vi "Strip prefix.vi"(10 "prefix":i32, 11 "address":refnum<class "IPv4 Network Address.lvclass">) -> (2 "subnet address":refnum<class "IPv4 Network Address.lvclass">)   [LabVIEW 2020, in "NI_WFCN.lvlib" / "IPv4 Network Address.lvclass"]
doc: "Masks the prefix off of this address, producing the subnet address. For instance, given address 192.168.1.2 and prefix 16, return 192.168.0.0."
uses:
  <vilib>/net/WFCN/Addressing/IPv4 Network Address/IPv4 Network Address.lvclass
  <vilib>/net/WFCN/Addressing/IPv4 Network Address/IPv4 Network Address.lvclass/IPv4 Network Address.ctl
  <vilib>/net/WFCN/NI_WFCN.lvlib
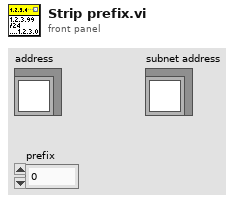
[diagram p1: front panel]
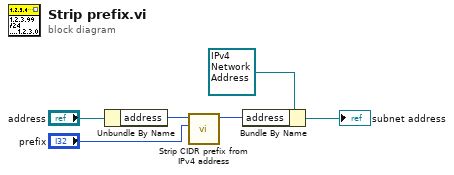
[diagram p0: block diagram]
diagram:
  n1 = Unbundle By Name("address") -> ("address"=w3:u32)
  n2 = call <vilib>:"Strip CIDR prefix from IPv4 address.vi"("prefix"="prefix", "address U32"=w3) -> ("address U32 out"=w1:u32)  [unwired: 9 in]
  n3 = Bundle By Name(cluster=refnum<class "IPv4 Network Address.lvclass"> refnum ("IPv4 Network Address in"), "address"=w1) -> (→"subnet address":refnum<class "IPv4 Network Address.lvclass">)
